vi "Util_GetTime_Orig.vi"(8 "error in (no error)":T1, 11 "Pass_Through_Time":numeric format="%33.4f") -> (0 "error out":T1, 2 "FPGA_Time_MicroSeconds":numeric format="%.0g", 3 "FPGA_Time_Seconds":numeric format="%33.4f")   [LabVIEW 2019]
doc: "This subVI returns the continuously running elapsed time in seconds. \n\nOn the RoboRIO this reads the high resolution FPGA time. The resolution, not accuracy, of the FPGA timer is 1 microsecond. The normal FPGA clock register (32 bits) rolls over approximately every 71 minutes. To significantly extend the rollover time,, this routine reads both the high and low FPGA clock registers. High/low register turnover read sequencing is dealt with by reading the high register twice, once before and once after the low register. If the values are different, the read is repeated to assure consistency between the high and low values. On a PC the standard operating system timer with 1 millisecond resolution is used. \n\nNotes:\n-------\n- On the RoboRIO this routine takes approximately 4.8 microseconds to execute. The WPI read FPGA clock routine takes approxmately 2.6 microseconds. The difference can be attributed to this routine reading to extra words from the FPGA. Each FPGA read takes approximately 1 microsecond. \n\n- Set a conditional complilation variable TRAJLIB_USEOSTIME and set it to a value of 1 to force this routine to read the RoboRIO operating system time instead of the FPGA time. This will have 1 millisecond resolution. This routine executes faster, approx 1 microsecond.\n\n - On the RoboRIO there is some drift between the FPGA and operating system clocks. The drift isn't consistent, but appears to be approximately 20 milliseconds / hour. This isn't enough to be of concern.\n\n\nInput parameters:\n - PassThroughTime -- double float -- If wired and the value is > 0 then this time is passed through and the FPGA time is not read. Allows calling functions to use a single time instant if desired.\n - Input Error -- Input error cluster\n\nReturns:\n - FPGA_Time_Seconds -- double float -- Elapsed time in seconds.\n - FPGA_Time_Microseconds -- Uint64 -- Elapsed time in microseconds (This can be used as an input to the Network Table routines to sychnronize times.)\n - Output Error -- Output error cluster. An error will be returned if there are problems reading the FPGA or of the FPGA clock high register changes twice while reading the value.\n\nCustom Errors:\n - 8020 -- The upper FPGA time register changed during both attempts to read the FPGA time values. The returned time may not be valid."
uses:
  <vilib>/Rock Robotics/SystemInterfaces/System/FPGA_SystemFRC FPGA Ref.ctl
  <vilib>/rvi/interface/nirviReadWriteControl/nirviReadWriteControl.xnode
  NiFpgaLv.dll
  <vilib>/Utility/error.llb/Error Cluster From Error Code.vi
  <vilib>/rvi/interface/Simulation/niFpgaSimulationCallBeginRW.vi
  <vilib>/rvi/errors/niLvFpgaAdjustHostInterfaceError.vi
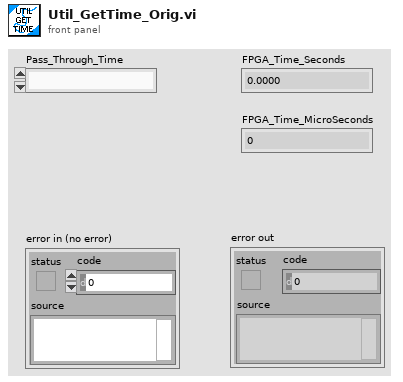
[diagram p1: front panel]
types:
  T1 = cluster{"source":string, "code":numeric, "status":boolean}
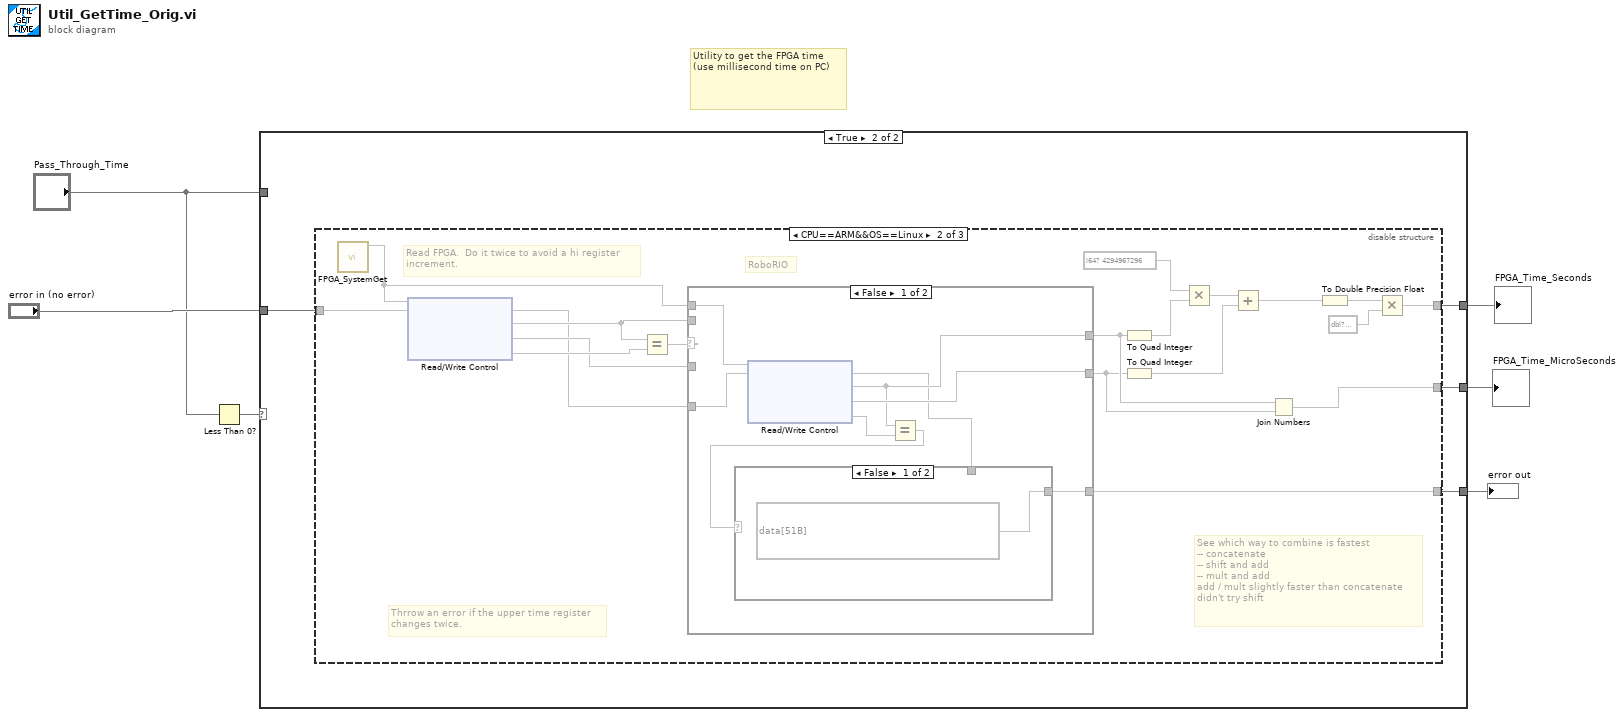
[diagram p0: block diagram]
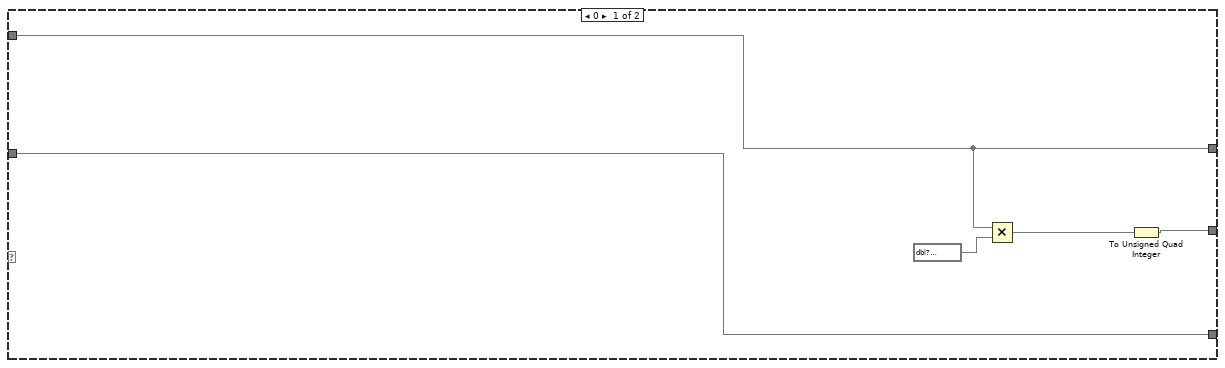
[diagram p2: hidden frame]
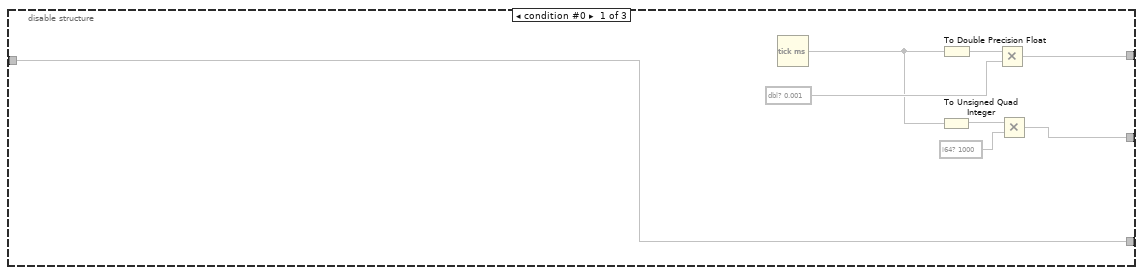
[diagram p3: hidden frame]
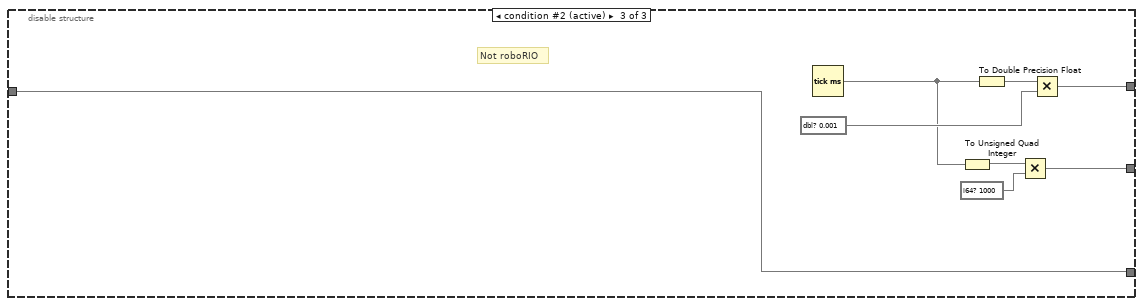
[diagram p6: hidden frame]
diagram:
  # "Utility to get the FPGA time\n(use millisecond time on PC)"
  n1 = Less Than 0?(x="Pass_Through_Time") -> (x < 0?=w3)
  n2 = case shown="True" w3 {
    tunnel: [w10 w15] -> w6
    tunnel: "error in (no error)" -> [w11 w14]
    tunnel: [w11 w13] -> w4
    tunnel: "Pass_Through_Time" -> [w10 _]
    tunnel: [w7 w12] -> w1
    frame 0 {
      n3 = Multiply(x=w10, y=dbl? 1000000.0) -> (x*y=w8)
      n4 = To Unsigned Quad Integer(1:w8) -> (0:w7)
    }
    frame 1 {
      n5 = disable-structure shown="CPU==ARM&&OS==Linux" {
        disable-tunnel: [w21 w40 w61] -> w15
        disable-tunnel: w14 -> [w20 w27 w60]
        disable-tunnel: [w20 w30 w60] -> w13
        disable-tunnel: [w16 w24 w56] -> w12
        frame condition #0 {
          n6 = Tick Count (ms)() -> (millisecond timer value=w19)
          n7 = To Unsigned Quad Integer(1:w19) -> (0:w18)
          n8 = To Double Precision Float(number=w19) -> (double precision float=w23)
          n9 = Multiply(x=w23, y=dbl? 0.001) -> (x*y=w21)
          n10 = Multiply(x=w18, y=i64? 1000) -> (x*y=w16)
        }
        frame condition #1 {
          # "See which way to combine is fastest\n-- concatenate\n-- shift and add\n-- mult and add\nadd / mult slightly faster than concatenate\ndidn't try shift"
          # "RoboRIO"
          # "Read FPGA.  Do it twice to avoid a hi register\nincrement."
          # "Thrrow an error if the upper time register\nchanges twice."
          n11 = call <vilib>:"FPGA_SystemGet.vi"() -> (3:w28)  [unwired: 11 in]
          n12 = xnode "Read/Write Control"(w28, w27) -> (w29, w32, w31, w39)  [unwired: 1 out]
          n13 = Equal?(x=w32, y=w39) -> (x = y?=w33)
          n14 = case shown="False" w33 {
            tunnel: [w47 w55] -> w26
            tunnel: w32 -> [_ w55]
            tunnel: [w48 w54] -> w25
            tunnel: w31 -> [_ w54]
            tunnel: [w44 w53] -> w30
            tunnel: w29 -> [w49 w53]
            tunnel: w28 -> [w50 _]
            frame 0 {
              n15 = xnode "Read/Write Control"(w50, w49) -> (w43, w47, w48, w46)  [unwired: 1 out]
              n16 = Equal?(x=w47, y=w46) -> (x = y?=w45)
              n17 = case shown="False" w45 {
                tunnel: [data[51B] ("error out") w52] -> w44
                tunnel: w43 -> [_ w52]
                frame 0 {
                }
                frame 1 {
                }
              }
            }
            frame 1 {
            }
          }
          n18 = To Quad Integer(1:w26) -> (0:w35)
          n19 = To Quad Integer(1:w25) -> (0:w34)
          n20 = Multiply(x=i64? 4294967296, y=w35) -> (x*y=w38)
          n21 = Add(x=w38, y=w34) -> (x+y=w36)
          n22 = Join Numbers(hi=w26, lo=w25) -> ((hi.lo)=w24)
          n23 = To Double Precision Float(number=w36) -> (double precision float=w41)
          n24 = Multiply(x=w41, y=dbl? 1e-06) -> (x*y=w40)
        }
        frame condition #2 (active) {
          # "Not roboRIO"
          n25 = Tick Count (ms)() -> (millisecond timer value=w57)
          n26 = To Unsigned Quad Integer(1:w57) -> (0:w59)
          n27 = To Double Precision Float(number=w57) -> (double precision float=w63)
          n28 = Multiply(x=w59, y=i64? 1000) -> (x*y=w56)
          n29 = Multiply(x=w63, y=dbl? 0.001) -> (x*y=w61)
        }
      }
    }
  }
  "FPGA_Time_Seconds" <- w6
  "error out" <- w4
  "FPGA_Time_MicroSeconds" <- w1
